vi "Get Cal Standard File Paths.vi"(11 "error in (no error)":errorcluster) -> (3 "Cal Standard Types":T1[](array[typedef]), 4 "Cal Standard File Paths":path[](array[path]), 6 "Found":bool, 15 "error out":errorcluster)   [LabVIEW 2023, in "Manual Cal Standard.lvlib" / "Cal Standard.lvclass"]
uses:
  Cal Standard.lvclass
  Instruments/Cal Standard/Type Definitions/Standard Type.ctl
  Utilities/Setting Keys.vi
  Common/Data Cache/Settings Dictionary/Setting Keys.vi
  Common/RFCalAndFixtureCharact.Common.lvlib
  Instruments/RFFixtureCharact.Instruments.lvlib
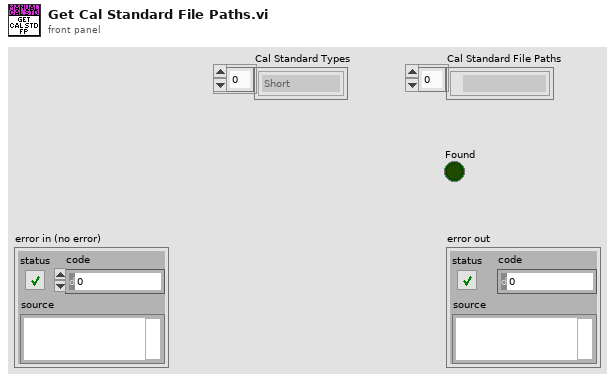
[diagram p1: front panel]
types:
  T1 = typedef "RFFixtureCharact.Instruments.lvlib/Standard Type.ctl" = enum16{"Short", "Open", "Load"}
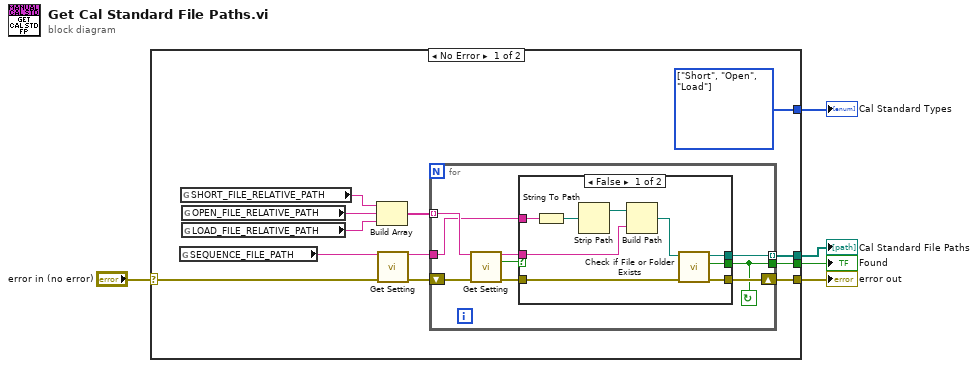
[diagram p0: block diagram]
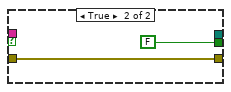
[diagram p2: hidden frame]
diagram:
  n1 = case shown="No Error" "error in (no error)" {
    selector: "error in (no error)" -> [w8 w38]
    tunnel: [w17 w38] -> w5
    tunnel: [w16 _] -> w4
    tunnel: [w7 _] -> w2
    tunnel: [w6 _] -> w1
    frame No Error {
      w6 = T1[] [enum."Short", enum."Open", enum."Load"] items=["Short", "Open", "Load"]
      n2 = global read "Setting Keys.vi" "SEQUENCE_FILE_PATH"() -> (w9:string)
      n3 = global read "Setting Keys.vi" "SHORT_FILE_RELATIVE_PATH"() -> (w11:string)
      n4 = global read "Setting Keys.vi" "OPEN_FILE_RELATIVE_PATH"() -> (w12:string)
      n5 = global read "Setting Keys.vi" "LOAD_FILE_RELATIVE_PATH"() -> (w13:string)
      n6 = Build Array(w11, w12, w13) -> (w14:string[])
      n7 = call "Get Setting.vi"("Setting name"=w9, "error in (no error)"=w8) -> ("Setting value out"=w15:string, "error out"=w10:errorcluster)  [unwired: 11 in, 1 out]
      n8 = for {
        shift-right: [w20] -> w17
        shift-left: w10 -> [w26]
        tunnel: w14 -> [w25] mode=indexing
        tunnel: w15 -> [w24]
        tunnel: [w19] -> w16 mode=indexing
        tunnel: [w18] -> w7
        stop <- w18 continue-if-true
        n9 = call "Get Setting.vi"("Setting name"=w25, "error in (no error)"=w26) -> ("Setting value out"=w21:string, "Setting empty or not found?"=w23:bool, "error out"=w22:errorcluster)  [unwired: 11 in]
        n10 = case shown="False" w23 {
          tunnel: w24 -> [w35 _]
          tunnel: w22 -> [w33 w37]
          tunnel: w21 -> [w34 _]
          tunnel: [w31 w37] -> w20
          tunnel: [w30 FALSE ("file or folder exists?")] -> w18
          tunnel: [w29 _] -> w19
          frame False {
            n11 = String To Path(string=w35) -> (path=w28:path)
            n12 = Strip Path(path=w28) -> (stripped path=w27:path)  [unwired: 1 out]
            n13 = Build Path(base path=w27, name or relative path=w34) -> (appended path=w32:path)
            n14 = call <vilib>:"Check if File or Folder Exists.vi"("error in (no error)"=w33, "path"=w32) -> ("error out"=w31:errorcluster, "file or folder exists?"=w30:bool, "dup path"=w29:path)  [unwired: 7 in]
          }
          frame True {
          }
        }
      }
    }
    frame Error {
    }
  }
  "error out" <- w5
  "Cal Standard File Paths" <- w4
  "Found" <- w2
  "Cal Standard Types" <- w1
